vi "BackTo.vi"(1 "Control in":T1={"queue"=refnum, "error"={"status"=FALSE, "code"=0, "source"=""}, "Step"={"Name"="", "Timeout"=0.0}, "Algorythm"=[{"Name"="Init", "Timeout"=0.0}]}, 9 "Back Step?":string) -> (15 "Control out":T1={"queue"=refnum, "error"={"status"=FALSE, "code"=0, "source"=""}, "Step"={"Name"="", "Timeout"=0.0}, "Algorythm"=[{"Name"="Init", "Timeout"=0.0}]})   [LabVIEW 2018, in "SFC.lvlib"]
uses:
  SFC.lvlib
  TypeDef/Control TypeDef.ctl
  TypeDef/Step TypeDef.ctl
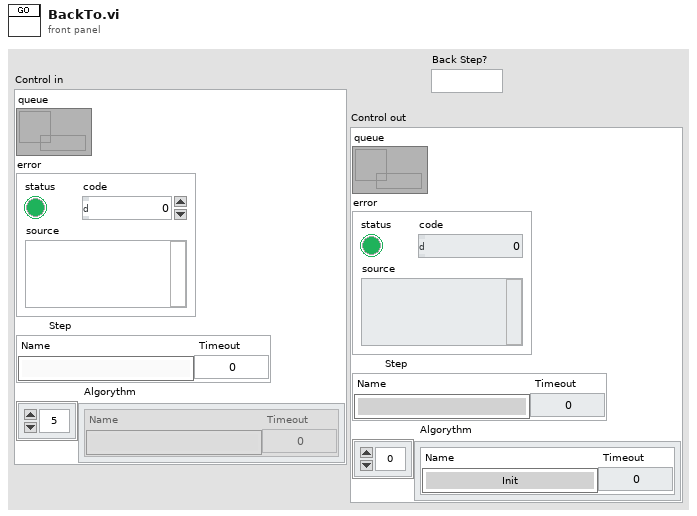
[diagram p1: front panel]
types:
  T1 = typedef "SFC.lvlib/Control TypeDef.ctl" = cluster{"queue":refnum<queue>, "error":errorcluster, "Step":T2, "Algorythm":T2[]}
  T2 = typedef "SFC.lvlib/Step TypeDef.ctl" = cluster{"Name":string, "Timeout":dbl}
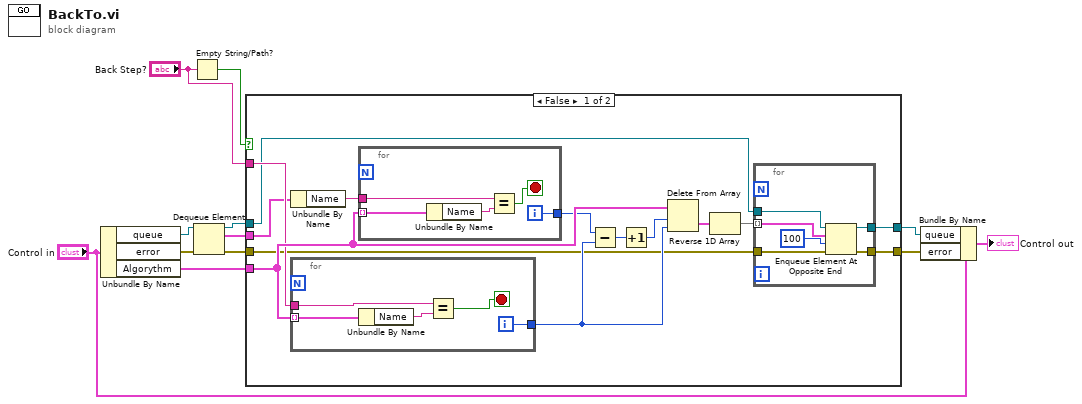
[diagram p0: block diagram]
diagram:
  n1 = Unbundle By Name("Control in") -> ("queue"=w7:refnum<queue>, "error"=w6:errorcluster, "Algorythm"=w2:T2[])
  n2 = Empty String/Path?(string/path="Back Step?") -> (empty?=w8:bool)
  n3 = Dequeue Element(queue=w7, error in (no error)=w6) -> (queue out=w4:refnum<queue>, element=w5:T2, error out=w3:errorcluster)  [unwired: 1 in, 1 out]
  n4 = case shown="False" w8 {
    tunnel: w2 -> [w26 _]
    tunnel: [w20 w44] -> w12
    tunnel: [w19 w43] -> w11
    tunnel: "Back Step?" -> [w17 _]
    tunnel: w5 -> [w16 _]
    tunnel: w4 -> [w14 w44]
    tunnel: w3 -> [w13 w43]
    frame False {
      n5 = Unbundle By Name(w16) -> ("Name"=w15:string)
      n6 = for {
        tunnel: w26 -> [w37] mode=indexing
        tunnel: w17 -> [w35]
        tunnel: [w33] -> w25
        i -> [w33]
        stop <- w34 stop-if-true
        n7 = Unbundle By Name(w37) -> ("Name"=w36:string)
        n8 = Equal?(x=w35, y=w36) -> (x = y?=w34:bool)
      }
      n9 = for {
        tunnel: w26 -> [w42] mode=indexing
        tunnel: w15 -> [w40]
        tunnel: [w38] -> w24
        i -> [w38]
        stop <- w39 stop-if-true
        n10 = Unbundle By Name(w42) -> ("Name"=w41:string)
        n11 = Equal?(x=w40, y=w41) -> (x = y?=w39:bool)
      }
      n12 = Subtract(x=w24, y=w25) -> (x-y=w23:i32)
      n13 = Increment(x=w23) -> (x+1=w22:i32)
      n14 = Delete From Array(array=w26, length=w22, index=w25) -> (deleted portion=w21:T2[])  [unwired: 1 out]
      n15 = Reverse 1D Array(array=w21) -> (reversed array=w18:T2[])
      n16 = for {
        tunnel: w14 -> [w32]
        tunnel: w13 -> [w31]
        tunnel: w18 -> [w29] mode=indexing
        tunnel: [w28] -> w20
        tunnel: [w27] -> w19
        n17 = Enqueue Element At Opposite End(queue=w32, element=w29, timeout in ms (-1)=100, error in (no error)=w31) -> (queue out=w28:refnum<queue>, error out=w27:errorcluster)  [unwired: 1 out]
      }
    }
    frame True {
    }
  }
  n18 = Bundle By Name(cluster="Control in", "queue"=w12, "error"=w11) -> (→"Control out":T1)
